vi "ReviewReports.vi"(5 "Q2Report":path=path "C:/Users/Min/Projects/SVN/Sniffer900/Server/AutoCal/Reference/Calibration Q2 Report150330 1500.jpg", 7 "Q1Report":path=path "C:/Users/Min/Projects/SVN/Sniffer900/Server/AutoCal/Reference/Calibration Q1 Report150330 1523.jpg") -> (3 "Accepted":bool=TRUE)   [LabVIEW 2015]
uses:
  Type/_RT Command.ctl
  <vilib>/Utility/NIReport.llb/Append Image to Report (path wrap).vi
  <vilib>/Utility/NIReport.llb/NI_report.lvclass
panel:
  in  "Exit":bool
  in  "Reject":bool
  in  "Accept":bool
  in  "Print":bool
  in  "Report To Review":u16(ring) items=["C:\\Users\\Min\\Projects\\SVN\\Sniffer900\\Server\\AutoCal\\Reference\\Calibration Q1 Report150330 1523.jpg", "C:\\Users\\Min\\Projects\\SVN\\Sniffer900\\Server\\AutoCal\\Reference\\Calibration Q2 Report150330 1500.jpg"]
  out "Report":picture
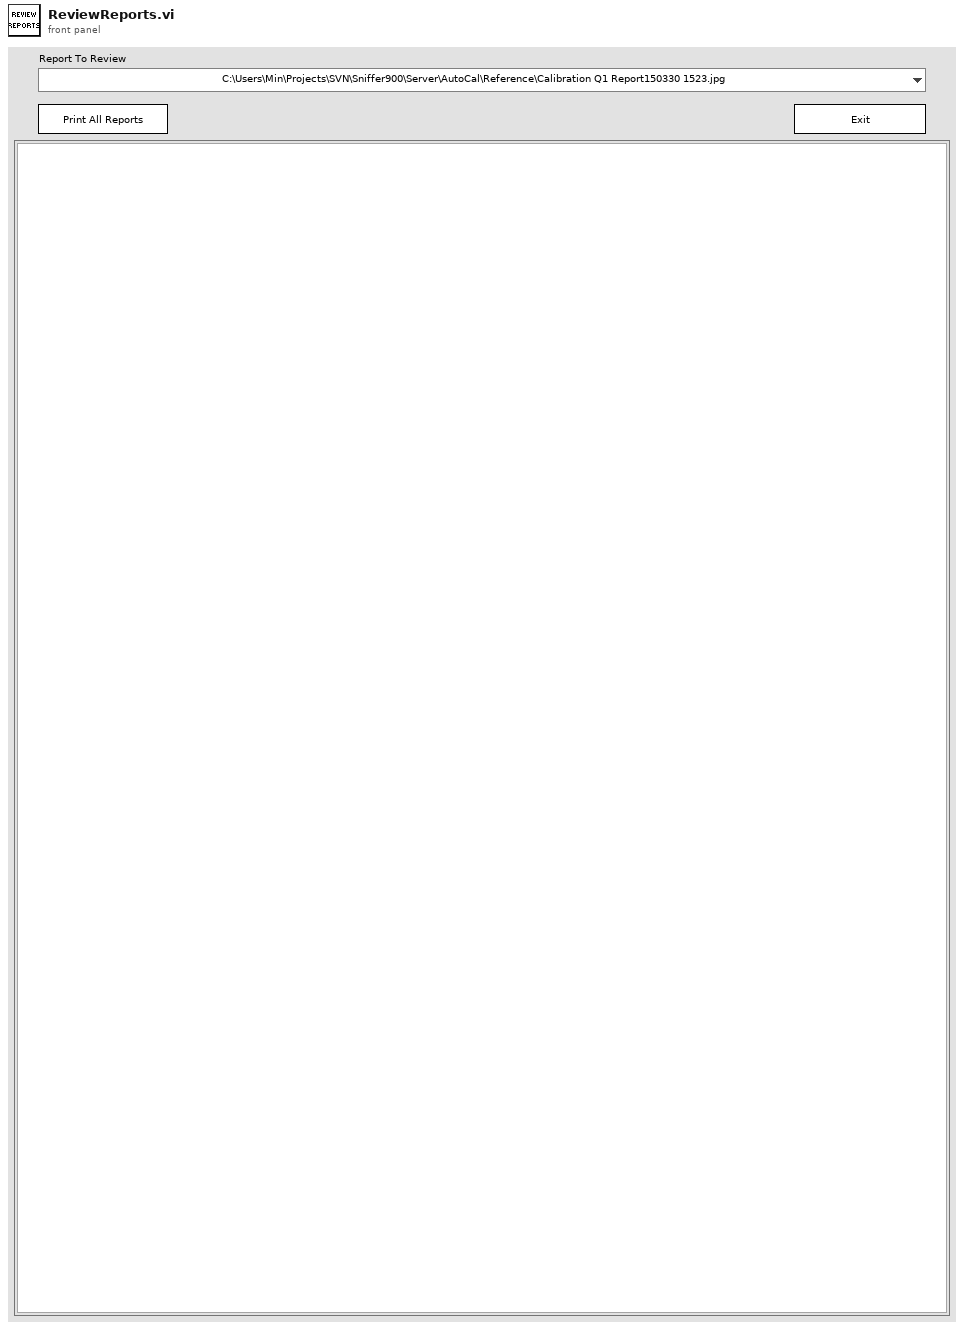
[diagram p1: front panel]
types:
  T1 = typedef "_RT Command.ctl" = enum16{"xml Start Run", "xml Start Actual Run", "xml Stop Run", "xml Runtime Update", "xml Get Status", "xml Get Table", "xml Set Table", "xml Get Configuration", "xml System Status", "xml Set LC Input Logic", "xml Get Data", "xml Get Info", "Start", "StartActualRun", "Stop", "Runtime Update", "Get Data", "Get Info", "Get Status", "Get Param", "Get Config", "Get Table", "Read ADC", "Set Oscillator", "Update Config", "Update Table", "Set All Pol", "Set Pol and DC", "Set Max Mass", "Toggle RP", "Toggle EL", "Set PIC", "Initialize Turbo", "Send Turbo Comm", "Close Turbo", "P1", "P2", "P3", "Send Serial", "Set LC Out", "Get LC In", "Read VAC", "Test Table", "Toggle Power", "Get Startup", "Set Startup", "Get ADC Table", "Set ADC Table", "Get Brief Status", "Get Detail Status", "Auxiliary Update", "Set CC Logics", "Set CC Input Logics", "Ignore Error", "invalid"}
  T2 = enum16{"Standard Report", "HTML", "Word", "Excel"}
  T3 = typedef "imagedata.ctl" = cluster{"image type":i32, "image depth":i32, "image":u8[], "mask":u8[], "colors":u32[], "Rectangle":cluster{"left":i16, "top":i16, "right":i16, "bottom":i16}}
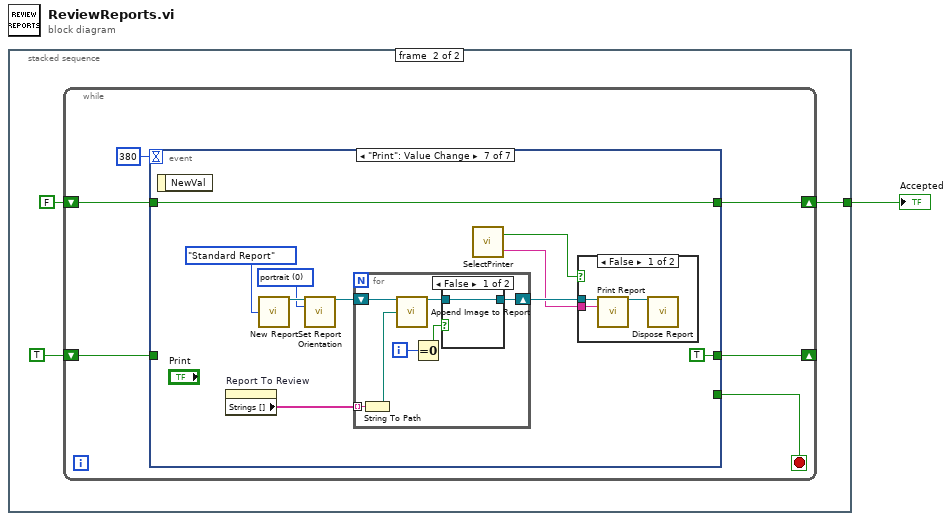
[diagram p0: block diagram]
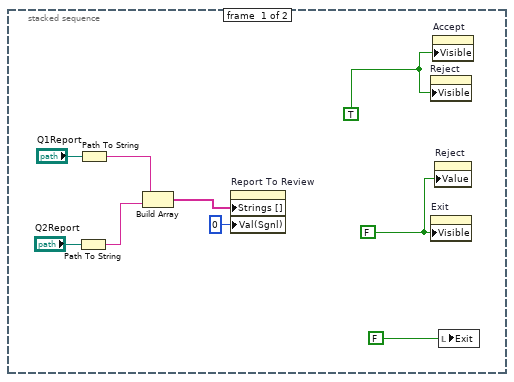
[diagram p2: hidden frame]
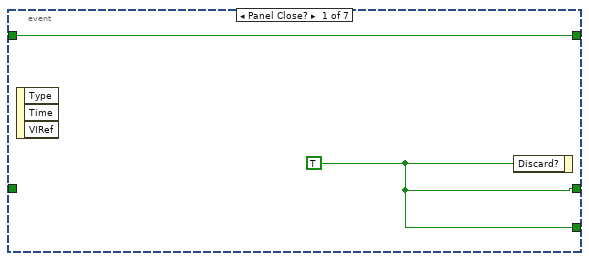
[diagram p3: hidden frame]
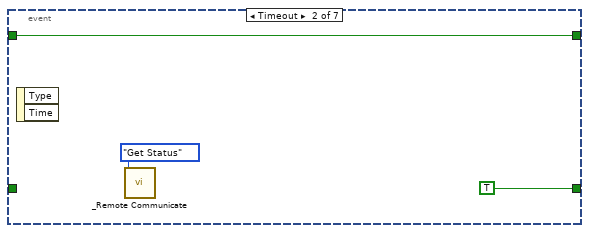
[diagram p4: hidden frame]
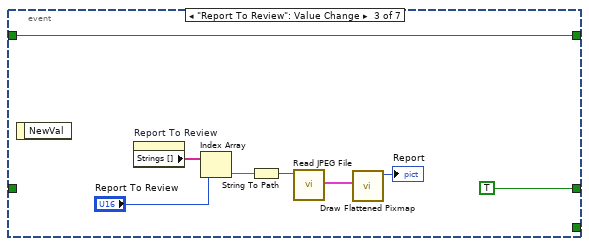
[diagram p5: hidden frame]
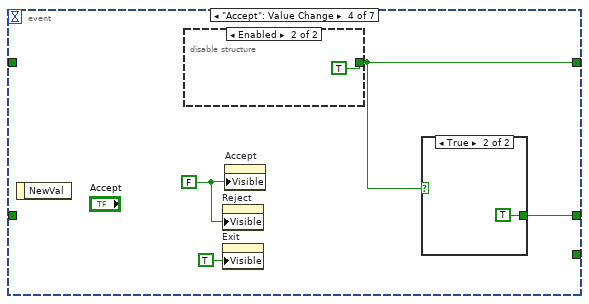
[diagram p6: hidden frame]
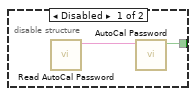
[diagram p7: hidden frame]
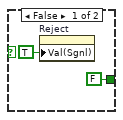
[diagram p8: hidden frame]
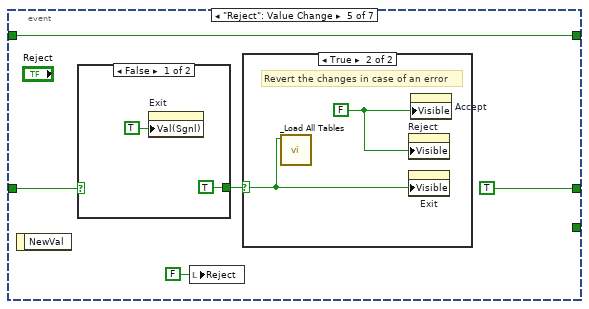
[diagram p9: hidden frame]
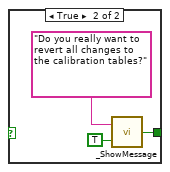
[diagram p10: hidden frame]
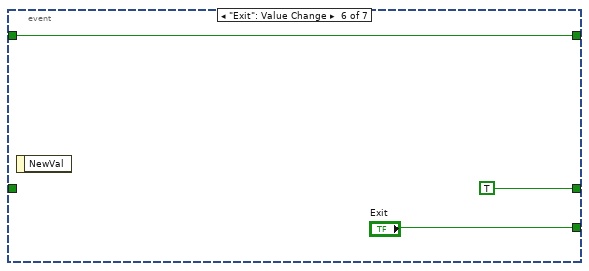
[diagram p12: hidden frame]
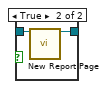
[diagram p14: hidden frame]
diagram:
  n1 = stacked-sequence {
    tunnel: [_ w12] -> w1
    frame #0 {
      w3 = FALSE ("Visible")
      w4 = TRUE ("Visible")
      n2 = Path To String(path="Q2Report") -> (string=w7:string)
      n3 = Path To String(path="Q1Report") -> (string=w8:string)
      n4 = Build Array(w8, w7) -> (w6:string[])
      n5 = property on="Report To Review" class="Ring (strict)"("Strings []"=w6, "Val(Sgnl)"=u16 0 ("Value (Signaling)")) -> ()  [unwired: 2 in, 2 out]
      n6 = property on="Reject" class="Bool (strict)"("Visible"=w4) -> ()  [unwired: 2 in, 2 out]
      n7 = property on="Exit" class="Bool (strict)"("Visible"=w3) -> ()  [unwired: 2 in, 2 out]
      n8 = property on="Accept" class="Bool"("Visible"=w4) -> ()  [unwired: 2 in, 2 out]
      n9 = property on="Reject" class="Bool (strict)"("Value"=w3) -> ()  [unwired: 2 in, 2 out]
      n10 = local write "Exit"(FALSE ("Exit")) -> ()
    }
    frame #1 {
      n11 = while {
        shift-right: [w16] -> _
        shift-left: TRUE ("TwoButton? (F)") -> [w17]
        shift-right: [w15] -> w12
        shift-left: FALSE ("Valid") -> [w14]
        stop <- w19 stop-if-true
        n12 = event shown="[6] \"Print\": Value Change" {
          selector: _ -> [_ _ _ _ _ _ _]
          dyn-events: _ -> [_ _ _ _ _ _ _]
          timeout: 380 -> [_ _ _ _ _ _ _]
          tunnel: [w21 _ _ _ _ "Exit" _] -> w19
          tunnel: w17 -> [_ _ _ _ w46 _ _]
          tunnel: [w21 TRUE ("Value (Signaling)") TRUE ("Value (Signaling)") w34 TRUE ("Value (Signaling)") TRUE ("Value (Signaling)") TRUE ("Value (Signaling)")] -> w16
          tunnel: [w20 w22 w25 w33 w43 w55 w58] -> w15
          tunnel: w14 -> [w20 w22 w25 _ w43 w55 w58]
          event Panel Close? {
            w21 = TRUE
            n13 = event-data() -> ()  [unwired: 1 in, 3 out]
            n14 = event-data("Discard?"=w21) -> ()  [unwired: 1 in, 1 out]
          }
          event Timeout {
            n15 = event-data() -> ()  [unwired: 1 in, 2 out]
            n16 = call "_Remote Communicate.vi"("Command"=_RT_Command."Get Status") -> ()  [unwired: 5 in, 4 out]
          }
          event "Report To Review": Value Change {
            n17 = event-data() -> ()  [unwired: 1 in, 1 out]
            n18 = property on="Report To Review" class="Ring (strict)"() -> ("Strings []"=w32:string[])  [unwired: 2 in, 2 out]
            n19 = Index Array(array=w32, index="Report To Review") -> (element=w30:string)
            n20 = String To Path(string=w30) -> (path=w27:path)
            n21 = call <vilib>:"Read JPEG File.vi"("path to JPEG file"=w27) -> ("image data"=w29:T3)  [unwired: 8 in, 2 out]
            n22 = call <vilib>:"Draw Flattened Pixmap.vi"("image data"=w29) -> ("new picture"=→"Report":picture)  [unwired: 8 in]
          }
          event "Accept": Value Change {
            w36 = FALSE ("Visible")
            n23 = event-data() -> ()  [unwired: 1 in, 1 out]
            n24 = disable-structure shown="Enabled" {
              disable-tunnel: [w37 TRUE ("Valid")] -> w33
              frame Disabled {
                n25 = call "Read AutoCal Password.vi"() -> ("Password"=w38:string)  [unwired: 10 in, 1 out]
                n26 = call "AutoCal Password.vi"("IonSniffer777"=w38) -> ("Valid"=w37:bool)  [unwired: 5 in, 1 out]
              }
              frame Enabled {
              }
            }
            n27 = property on="Reject" class="Bool (strict)"("Visible"=w36) -> ()  [unwired: 2 in, 2 out]
            n28 = property on="Exit" class="Bool (strict)"("Visible"=TRUE) -> ()  [unwired: 2 in, 2 out]
            n29 = property on="Accept" class="Bool"("Visible"=w36) -> ()  [unwired: 2 in, 2 out]
            n30 = case shown="True" w33 {
              tunnel: [FALSE ("Value (Signaling)") TRUE ("Value (Signaling)")] -> w34
              frame False {
                n31 = property on="Reject" class="Bool (strict)"("Val(Sgnl)"=TRUE ("Value (Signaling)")) -> ()  [unwired: 2 in, 2 out]
              }
              frame True {
              }
            }
          }
          event "Reject": Value Change {
            n32 = event-data() -> ()  [unwired: 1 in, 1 out]
            n33 = case shown="False" w46 {
              tunnel: [TRUE ("Ok?") w51] -> w47
              frame False {
                n34 = property on="Exit" class="Bool (strict)"("Val(Sgnl)"=TRUE ("Value (Signaling)")) -> ()  [unwired: 2 in, 2 out]
              }
              frame True {
                n35 = call "_ShowMessage.vi"("TwoButton? (F)"=TRUE, "Message"="Do you really want to revert all changes to the calibration tables?" ("message")) -> ("Ok?"=w51:bool)
              }
            }
            n36 = local write "Reject"(FALSE ("Reject")) -> ()
            n37 = case shown="True" w47 {
              selector: w47 -> [_ w54]
              frame False {
              }
              frame True {
                w53 = FALSE ("Use temporary file (F)")
                # "Revert the changes in case of an error"
                n38 = call "_Load All Tables.vi"("Use temporary file (F)"=w54) -> ()  [unwired: 7 out]
                n39 = property on="Reject" class="Bool (strict)"("Visible"=w53) -> ()  [unwired: 2 in, 2 out]
                n40 = property on="Exit" class="Bool (strict)"("Visible"=w54) -> ()  [unwired: 2 in, 2 out]
                n41 = property on="Accept" class="Bool"("Visible"=w53) -> ()  [unwired: 2 in, 2 out]
              }
            }
          }
          event "Exit": Value Change {
            n42 = event-data() -> ()  [unwired: 1 in, 1 out]
          }
          event "Print": Value Change {
            w63 = 0 items=["portrait", "landscape"] ("orientation (portrait)")
            n43 = event-data() -> ()  [unwired: 1 in, 1 out]
            n44 = property on="Report To Review" class="Ring (strict)"() -> ("Strings []"=w67:string[])  [unwired: 2 in, 2 out]
            n45 = call <vilib>:"New Report.vi"("report type"=T2."Standard Report") -> ("report out"=w64:refnum<class "NI_report.lvclass">)  [unwired: 13 in, 1 out]
            n46 = call-dynamic "Set Report Orientation.vi"("report in"=w64, "orientation (portrait)"=w63) -> ("report out"=w61:refnum<class "NI_report.lvclass">)  [unwired: 12 in, 1 out]
            n47 = for {
              tunnel: w67 -> [w77] mode=indexing
              shift-right: [w73] -> w65
              shift-left: w61 -> [w76]
              i -> [w71]
              n48 = String To Path(string=w77) -> (path=w75:path)
              n49 = call-poly <vilib>:"Append Image to Report.vi"("report in"=w76, "path or URL of image"=w75) -> ("report out"=w74:refnum<class "NI_report.lvclass">)  [unwired: 10 in, 3 out]
              n50 = Equal To 0?(x=w71) -> (x = 0?=w72:bool)
              n51 = case shown="False" w72 {
                tunnel: w74 -> [w78 w80]
                tunnel: [w78 w79] -> w73
                frame False {
                }
                frame True {
                  n52 = call-dynamic "New Report Page.vi"("report in"=w80) -> ("report out"=w79:refnum<class "NI_report.lvclass">)  [unwired: 13 in, 1 out]
                }
              }
            }
            n53 = call "SelectPrinter.vi"() -> ("ChosenPrinter"=w62:string, "Closed?"=w59:bool)  [unwired: 2 in]
            n54 = case shown="False" w59 {
              tunnel: w65 -> [w70 _]
              tunnel: w62 -> [w68 _]
              frame False {
                n55 = call-dynamic "Print Report.vi"("report in"=w70, "printer name (default)"=w68) -> ("report out"=w69:refnum<class "NI_report.lvclass">)  [unwired: 12 in, 1 out]
                n56 = call-dynamic "Dispose Report.vi"("report in"=w69) -> ()  [unwired: 14 in, 1 out]
              }
              frame True {
              }
            }
          }
        }
      }
    }
  }
  "Accepted" <- w1
